vi "ReadData.vi"(8 "Error In":errorcluster, 11 "Connection In":refnum<k5>) -> (0 "Error Out":errorcluster, 2 "Data Out":u8[](array[numeric]), 3 "Connection Out":refnum<k5>)   [LabVIEW 2019]
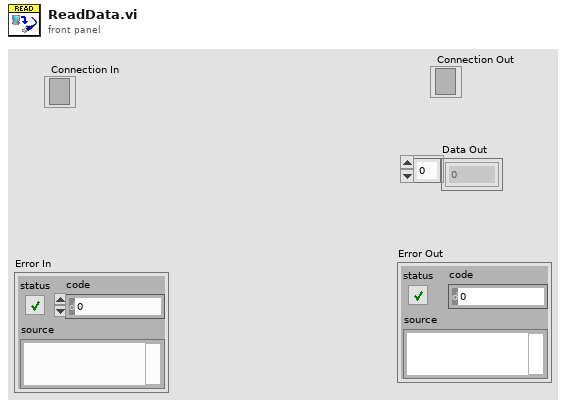
[diagram p1: front panel]
types:
  T1 = enum16{"big-endian, network order", "native, host order", "little-endian"}
  T2 = enum16{"Standard", "Buffered", "CRLF", "Immediate"}
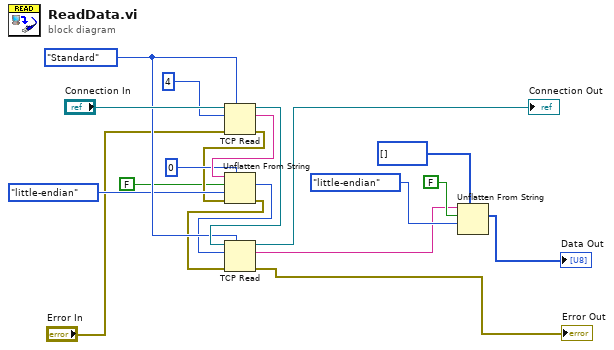
[diagram p0: block diagram]
diagram:
  w14 = T2."Standard" ("mode (standard)")
  n1 = TCP Read(connection ID="Connection In", bytes to read=4, error in (no error)="Error In", 7:w14) -> (connection ID out=w15:refnum<k5>, data out=w17:string, error out=w9:errorcluster)  [unwired: 1 in]
  n2 = Unflatten From String(type=0, binary string=w17, data includes array or string size? (T)=FALSE, byte order (0:big-endian, network order)=T1."little-endian", error in (no error)=w9) -> (value=w13:i32, error out=w8:errorcluster)  [unwired: 1 out]
  n3 = TCP Read(connection ID=w15, bytes to read=w13, error in (no error)=w8, 7:w14) -> (connection ID out=→"Connection Out":refnum<k5>, data out=w3:string, error out=→"Error Out":errorcluster)  [unwired: 1 in]
  n4 = Unflatten From String(type=u8[] [], binary string=w3, data includes array or string size? (T)=FALSE, byte order (0:big-endian, network order)=T1."little-endian") -> (value=→"Data Out":u8[])  [unwired: 1 in, 2 out]
